vi "get State.vi"(11 "Blinker in":refnum<class "Blinker.lvclass">) -> (3 "Blink State":bool)   [LabVIEW 2015, in "Blinker.lvclass"]
uses:
  Blinker.lvclass
  Blinker.lvclass/Blinker.ctl
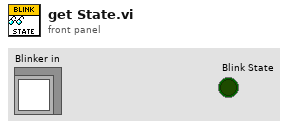
[diagram p1: front panel]
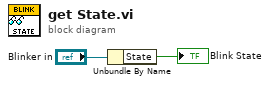
[diagram p0: block diagram]
diagram:
  n1 = Unbundle By Name("Blinker in") -> ("State"=→"Blink State":bool)
